vi "Exp_Setup_Control.vi"(2 "Dispersion?":bool) -> ()   [LabVIEW 2015]
uses:
  ADAM Controls/Channel_State.ctl
  Anemometry/Anemometry Sub Vis/Globals/Preference_global.vi
  Anemometry/Anemometry Sub Vis/Globals/Trav_pos_global.vi
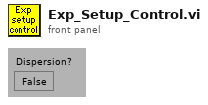
[diagram p1: front panel]
types:
  T1 = typedef "Channel_State.ctl" = enum16{"On", "Off", "Always On", "Always Off"}
  T2 = typedef "Ch_description_ADAM.ctl" = cluster{"Ch Name":string, "Type":T3, "Function":T4, "Ch State":T1, "Calibration type":T5, "A":dbl, "B":dbl, "C":dbl, "D":dbl, "Comments":string, "Address":T6, "String":string, "Duty":u16}
  T3 = typedef "Module_type_ADAM.ctl" = string
  T4 = typedef "Function_ADAM.ctl" = enum16{"Analogue Input", "Digital Input", "Event counter", "Event rate", "Analogue Output", "Digital Output", "Relay Output"}
  T5 = typedef "Calib_type_ADAM.ctl" = enum16{"Raw", "Bx + A", "Cx^2 + Bx + A", "Dx^3 + Cx^2 + Bx + A", "In Band", "Hi-Tec Q", "Hi-Tec M_dot", "Text"}
  T6 = typedef "Address.ctl" = cluster{"Main":i32, "Ch.":i32, "Sub":i32, "Port Name":string}
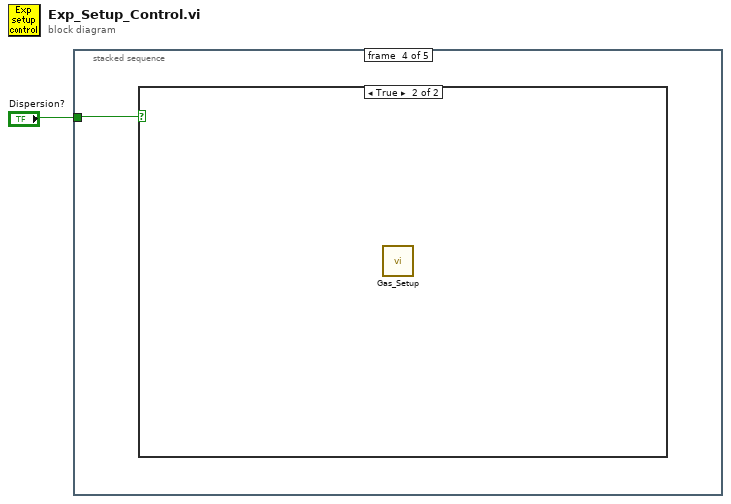
[diagram p0: block diagram]
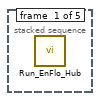
[diagram p2: hidden frame]
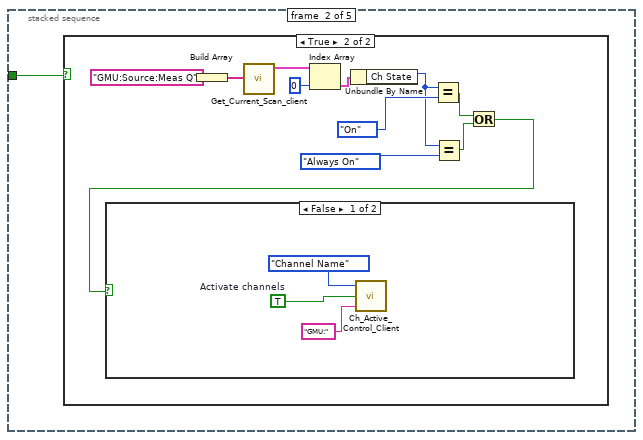
[diagram p3: hidden frame]
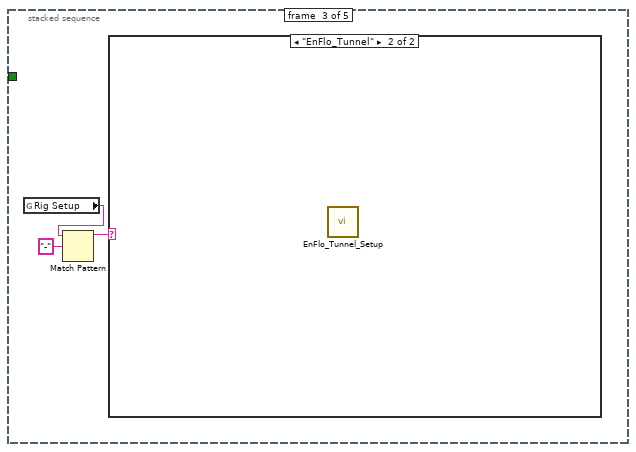
[diagram p6: hidden frame]
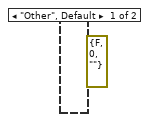
[diagram p7: hidden frame]
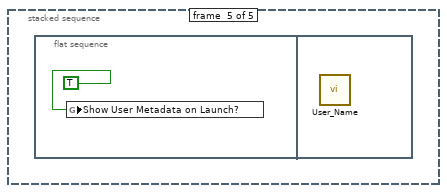
[diagram p9: hidden frame]
diagram:
  n1 = stacked-sequence {
    tunnel: "Dispersion?" -> [_ w2 _ w20 _]
    frame #0 {
      n2 = call "Run_EnFlo_Hub.vi"() -> ()  [unwired: 8 out]
    }
    frame #1 {
      n3 = case shown="True" w2 {
        frame False {
        }
        frame True {
          n4 = Build Array("GMU:Source:Meas Q") -> (w12:string[])
          n5 = call "Get_Current_Scan_client.vi"("ADAM Ch Names"=w12) -> ("Ch Description Array"=w11:T2[])  [unwired: 3 out]
          n6 = Index Array(array=w11, index=0 ("Index")) -> (element=w9:T2)
          n7 = Unbundle By Name(w9) -> ("Ch State"=w7:T1)
          n8 = Equal?(x=w7, y=Channel_State."On" ("Channel State")) -> (x = y?=w4:bool)
          n9 = Equal?(x=w7, y=Channel_State."Always On" ("Channel State")) -> (x = y?=w5:bool)
          n10 = Or(x=w4, y=w5) -> (x .or. y?=w3:bool)
          n11 = case shown="False" w3 {
            frame False {
              w14 = TRUE  # Activate channels
              n12 = call "Ch_Active_Control_Client.vi"("Match"="GMU:", "Activate Channels?"=w14, "Control on"=enum16{"Channel Name", "Main Address"}."Channel Name") -> ()  [unwired: 2 out]
            }
            frame True {
            }
          }
        }
      }
    }
    frame #2 {
      n13 = global read "Preference_global.vi" "Rig Setup"() -> (w18:string)
      n14 = Match Pattern(string=w18, regular expression="-") -> (before substring=w17:string)  [unwired: 4 out]
      n15 = case shown="\"EnFlo_Tunnel\"" w17 {
        frame "Other", Default {
          (unwired) errorcluster {"status"=FALSE, "code"=0, "source"=""} ("error out")
        }
        frame "EnFlo_Tunnel" {
          n16 = call "EnFlo_Tunnel_Setup.vi"() -> ()  [unwired: 9 out]
        }
      }
    }
    frame #3 {
      n17 = case shown="True" w20 {
        frame False {
        }
        frame True {
          n18 = call "Gas_Setup.vi"() -> ()  [unwired: 9 out]
        }
      }
    }
    frame #4 {
      n19 = flat-sequence {
        frame #0 {
          n20 = global write "Trav_pos_global.vi" "Show User Metadata on Launch?"(TRUE) -> ()
        }
        frame #1 {
          n21 = call "User_Name.vi"() -> ()  [unwired: 1 out]
        }
      }
    }
  }
